vi "Read_Joint_States.vi"   [LabVIEW 2013]
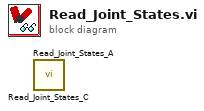
[diagram p0: block diagram]
diagram:
  n1 = call "Read_Joint_States_C.vi"() -> ()  [unwired: 5 in, 4 out]
  n2 = call "Read_Joint_States_A.vi"() -> ()  [unwired: 5 in, 4 out]
